vi "IMAQdx_grab_att - Kopie.vi"() -> ()   [LabVIEW 2015]
doc: "The Grab VI acquires images continuously and displays the images in an image control using low-level acquisition VIs. A grab is appropriate for high-speed applications in which you need to process only one image at a time."
uses:
  <vilib>/userdefined/High Color/IMAQdx.ctl
  <vilib>/vision/driver/IMAQdx.llb/IMAQdx Attribute Type.ctl
  <vilib>/vision/driver/IMAQdx.llb/IMAQdx Acquisition Mode.ctl
  <vilib>/vision/driver/IMAQdx.llb/IMAQdx Buffer Number Mode.ctl
  <vilib>/vision/driver/NI_Vision_Acquisition_Software.lvlib
  <resource>/objmgr/imaqdx.rc
  <vilib>/vision/NI_Vision_Development_Module.lvlib
panel:
  out "Exposure::Mode 2":u32(ring)=2 caption="Exposure::Mode" items=["Auto"=1, "Manual"=2]
  in  "String":string="um"
  out "output cluster":cluster{sgl, sgl}
  out "Last Mouse Position:All Elements":cluster{"X":i32, "Y":i32}
  in  "Gain::Value":i64 min=0 max=1728 step=1
  in  "Gain::Mode":u32(ring)=2 items=["Auto"=1, "Manual"=2]
  in  "Exposure::Value":dbl=0.0625 min=0.0 max=0.125
  in  "Exposure::Mode":u32(ring)=2 items=["Auto"=1, "Manual"=2]
  in  "Pixel Distances":T1={"X Step"=5.2, "Y Step"=5.2, "Unit"=enum."Micrometer"} {"Y Step" format="%.2f"; "X Step" format="%.2f"}
  out "Image Pixels (U8)":u8[][](array[numeric])
  out "error out":errorcluster
  out "Luminance Plane":T3(plugin-control)
  out "MinDBL":dbl
  out "MaxDBL":dbl
  out "Units":string
  in  "SetExpMode":enum16{"Dont use this!", "Auto", "Manual"}(ring)=enum."Auto"
  out "GetExpVal":dbl
  out "Attribute Information Array":T5(array[cluster])
  in  "InitExpVal":dbl
  out "IMAQdx Session":T6
  in  "Camera Name":refnum<k21>="cam0" caption="IMAQdx Session"
  out "Buffer Number":u32
  out "Image":T3(plugin-control)
  out "Frame Rate":dbl(knob) scale=0.0..20.0
  in  "Stop":bool
  # "Overview: Demonstrates how to acquire continuous images from a camera using low level acquisition functions.\nRequirements: Vision Acquisition Software\nInstructions:\n1. Select the Camera Name\n2. Run the VI"
  # "x /µm"
  # "y /µm"
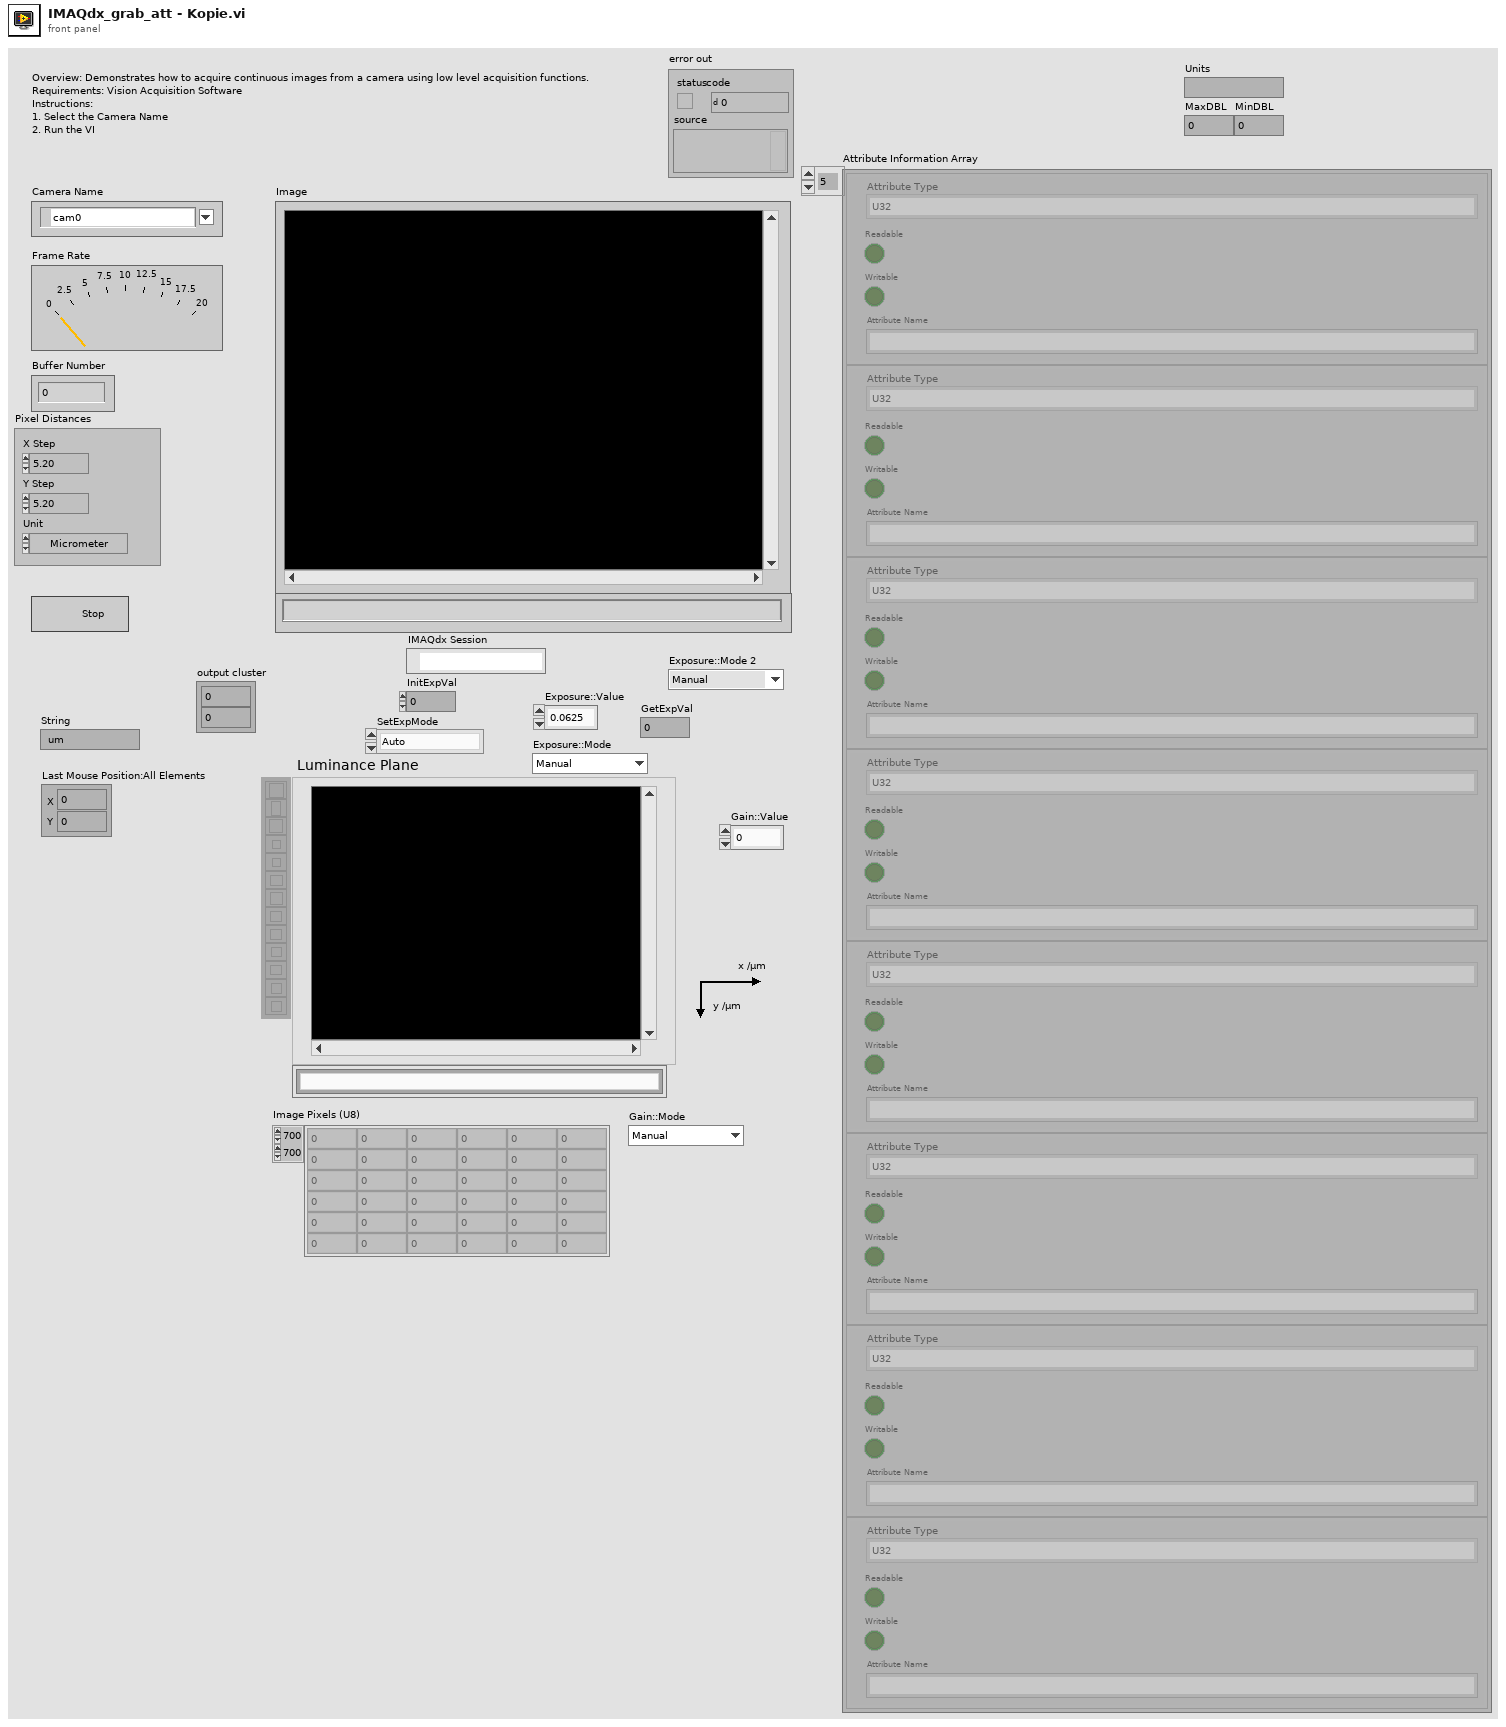
[diagram p1: front panel]
types:
  T1 = typedef "Simple Grid Descriptor" = cluster{"X Step":sgl, "Y Step":sgl, "Unit":T2}
  T2 = typedef "Image Unit" = enum32{"Undefined", "Angström", "Micrometer", "Millimeter", "Centimeter", "Meter", "Kilometer", "Microinch", "Inch", "Feet", "Nautical miles", "Standard miles", "Steps"}
  T3 = typedef "IMAQ Image.ctl" = refnum<image>
  T4 = typedef "NI_Vision_Acquisition_Software.lvlib/IMAQdx Attribute Type.ctl" = enum32{"U32", "I64", "DBL", "String", "Enum", "Bool", "Command"}
  T5 = cluster{"Attribute Type":T4, "Readable":bool, "Writable":bool, "Attribute Name":string}[]
  T6 = typedef "IMAQdx.ctl" = refnum<k21>
  T7 = typedef "Image Type" = u32
  T8 = typedef "NI_Vision_Acquisition_Software.lvlib/IMAQdx Acquisition Mode.ctl" = enum32{"One Shot", "Continuous"}
  T9 = typedef "NI_Vision_Acquisition_Software.lvlib/IMAQdx Buffer Number Mode.ctl" = enum32{"Next", "Last", "Buffer Number", "Every", "Last New"}
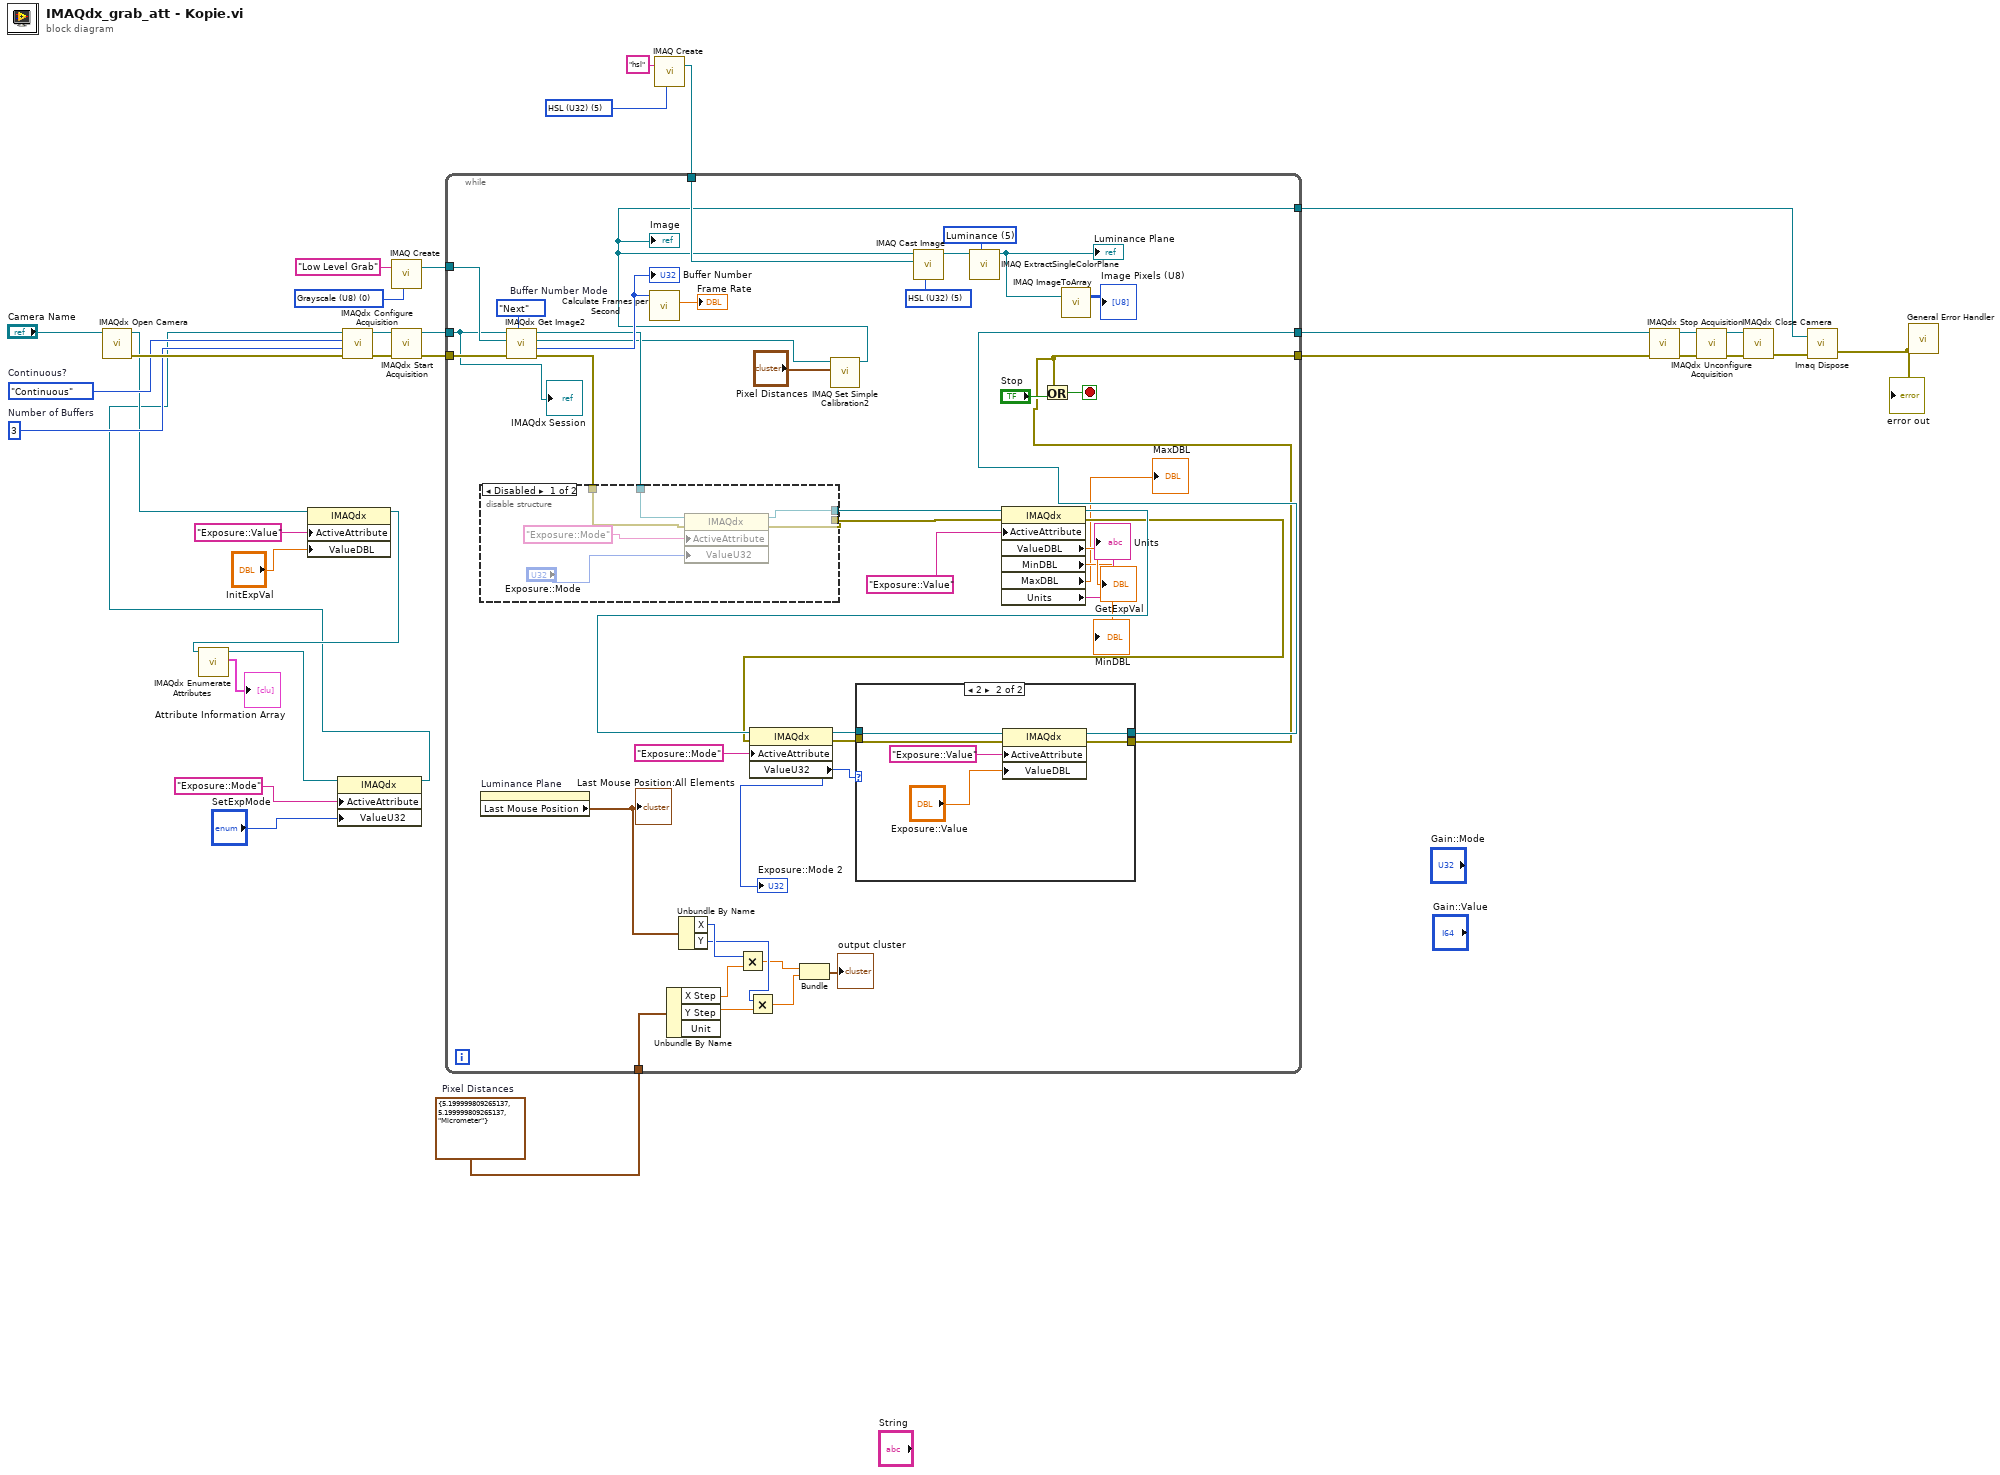
[diagram p0: block diagram]
diagram:
  w1 = T1 {"X Step"=5.2, "Y Step"=5.2, "Unit"=enum."Micrometer"}  # Pixel Distances
  w8 = T7 5 items=["Grayscale (U8)", "Grayscale (I16)", "Grayscale (SGL)", "Complex (CSG)", "RGB (U32)", "HSL (U32)", "RGB (U64)"] ("Image Type")
  w10 = T7 0 items=["Grayscale (U8)", "Grayscale (I16)", "Grayscale (SGL)", "Complex (CSG)", "RGB (U32)", "HSL (U32)", "RGB (U64)", "Grayscale (U16)"] ("Image Type")
  w26 = u32 3  # Number of Buffers
  w27 = IMAQdx_Acquisition_Mode."Continuous"  # Continuous?
  n1 = call <vilib>:"IMAQdx Open Camera.vi"("Session In"="Camera Name") -> ("error out"=w30:errorcluster, "Session Out"=w15:T6)  [unwired: 2 in, 7 out]
  n2 = property class="IMAQdx"(reference=w15, "ActiveAttribute"="Exposure::Value", "ValueDBL"="InitExpVal") -> (reference out=w12:T6)  [unwired: 1 in, 1 out]
  n3 = call <vilib>:"IMAQdx Enumerate Attributes.vi"("Session In"=w12) -> ("Attribute Information Array"=→"Attribute Information Array":T5, "Session Out"=w5:T6)  [unwired: 8 in, 1 out]
  n4 = property class="IMAQdx"(reference=w5, "ActiveAttribute"="Exposure::Mode", "ValueU32"="SetExpMode") -> (reference out=w4:T6)  [unwired: 1 in, 1 out]
  n5 = call <vilib>:"IMAQdx Configure Acquisition.vi"("error in"=w30, "Number of Buffers"=w26, "Continuous?"=w27, "Session In"=w4) -> ("error out"=w29:errorcluster, "Session Out"=w31:T6)  [unwired: 6 out]
  n6 = call "IMAQ Create"("Image Name"="Low Level Grab", "Image Type"=w10) -> ("New Image"=w33:T3)  [unwired: 2 in, 2 out]
  n7 = call <vilib>:"IMAQdx Start Acquisition.vi"("error in"=w29, "Session In"=w31) -> ("error out"=w28:errorcluster, "Session Out"=w2:T6)  [unwired: 8 out]
  n8 = call "IMAQ Create"("Image Name"="hsl", "Image Type"=w8) -> ("New Image"=w7:T3)  [unwired: 3 in, 1 out]
  n9 = while {
    tunnel: [w63] -> w24
    tunnel: w28 -> [w75]
    tunnel: w2 -> [w69]
    tunnel: [w62] -> w25
    tunnel: w33 -> [w74]
    tunnel: [w47] -> w16
    tunnel: w7 -> [w50]
    tunnel: w1 -> [w44]
    stop <- w76 stop-if-true
    w52 = 5 items=["Red", "Green", "Blue", "Hue", "Saturation", "Luminance", "Value", "Intensity"] ("Color Plane")
    w53 = T7 5 items=["Grayscale (U8)", "Grayscale (I16)", "Grayscale (SGL)", "Complex (CSG)", "RGB (U32)", "HSL (U32)", "RGB (U64)"] ("Image Type")
    w72 = IMAQdx_Buffer_Number_Mode."Next"  # Buffer Number Mode
    n10 = property on="Luminance Plane" class="ImageControl"() -> ("Last Mouse Position"=w43:cluster{"X":i32, "Y":i32})  [unwired: 2 in, 2 out]
    "Last Mouse Position:All Elements" <- w43
    n11 = call <vilib>:"IMAQdx Get Image2.vi"("Buffer Number Mode (Next)"=w72, "error in"=w75, "Image In"=w74, "Session In"=w69) -> ("error out"=w65:errorcluster, "Buffer Number Out"=w71:u32, "Image Out"=w46:T3, "Session Out"=w64:T6)  [unwired: 4 in]
    "Buffer Number" <- w71
    n12 = disable-structure shown="Disabled" {
      disable-tunnel: [w81 w84] -> w67
      disable-tunnel: [w80 w83] -> w66
      disable-tunnel: w65 -> [w79 w83]
      disable-tunnel: w64 -> [w78 w84]
      frame Disabled {
        n13 = property class="IMAQdx"(reference=w78, error in=w79, "ActiveAttribute"="Exposure::Mode", "ValueU32"="Exposure::Mode") -> (reference out=w81:T6, error out=w80:errorcluster)
      }
      frame Enabled {
      }
    }
    n14 = call <vilib>:"Calculate Frames per Second.vi"("Buffer Number"=w71) -> ("Processed Frames/s"=→"Frame Rate":dbl)  [unwired: 8 in, 2 out]
    n15 = Unbundle By Name(w44) -> ("X Step"=w41:sgl, "Y Step"=w39:sgl)  [unwired: 1 out]
    n16 = Unbundle By Name(w43) -> ("X"=w42:i32, "Y"=w40:i32)
    n17 = Multiply(x=w42, y=w41) -> (x*y=w37:sgl)
    n18 = Multiply(x=w40, y=w39) -> (x*y=w38:sgl)
    n19 = Bundle(w37, w38) -> (→"output cluster":cluster{sgl, sgl})  [unwired: 1 in]
    n20 = call "IMAQ Set Simple Calibration2"("Pixel Distances"="Pixel Distances", "Image"=w46) -> ("Calibration Template Image"=w47:T3)  [unwired: 8 in, 1 out]
    "Image" <- w47
    n21 = call "IMAQ Cast Image"("Image Type"=w53, "Image Dst"=w50, "Image Src"=w47) -> ("Image Dst Out"=w51:T3)  [unwired: 7 in, 1 out]
    n22 = call "IMAQ ExtractSingleColorPlane"("Color Plane"=w52, "Image Src"=w51) -> ("Image Dst Out"=w45:T3)  [unwired: 8 in, 1 out]
    "Luminance Plane" <- w45
    n23 = property class="IMAQdx"(reference=w67, error in=w66, "ActiveAttribute"="Exposure::Value") -> (reference out=w59:T6, error out=w58:errorcluster, "ValueDBL"=→"GetExpVal":dbl, "MinDBL"=→"MinDBL":dbl, "MaxDBL"=→"MaxDBL":dbl, "Units"=→"Units":string)
    n24 = property class="IMAQdx"(reference=w59, error in=w58, "ActiveAttribute"="Exposure::Mode") -> (reference out=w57:T6, error out=w56:errorcluster, "ValueU32"=w34:u32)
    "Exposure::Mode 2" <- w34
    n25 = case shown="2" w34 {
      tunnel: w57 -> [w86 w91]
      tunnel: w56 -> [w85 w90]
      tunnel: [w86 w89] -> w63
      tunnel: [w85 w88] -> w62
      frame 1, Default {
      }
      frame 2 {
        n26 = property class="IMAQdx"(reference=w91, error in=w90, "ActiveAttribute"="Exposure::Value", "ValueDBL"="Exposure::Value") -> (reference out=w89:T6, error out=w88:errorcluster)
      }
    }
    n27 = Or(x=w62, y="Stop") -> (x .or. y?=w76:bool)
    n28 = call "IMAQ ImageToArray"("Image"=w45) -> ("Image Pixels (U8)"=→"Image Pixels (U8)":u8[][])  [unwired: 3 in, 4 out]
    "IMAQdx Session" <- w69
  }
  n29 = call <vilib>:"IMAQdx Stop Acquisition.vi"("error in"=w25, "Session In"=w24) -> ("error out"=w20:errorcluster, "Session Out"=w21:T6)  [unwired: 8 out]
  n30 = call <vilib>:"IMAQdx Unconfigure Acquisition.vi"("error in"=w20, "Session In"=w21) -> ("error out"=w23:errorcluster, "Session Out"=w22:T6)  [unwired: 8 out]
  n31 = call <vilib>:"IMAQdx Close Camera.vi"("error in"=w23, "Session In"=w22) -> ("error out"=w19:errorcluster)  [unwired: 9 out]
  n32 = call "Imaq Dispose"("Image"=w16, "error in (no error)"=w19) -> ("error out"=w18:errorcluster)  [unwired: 4 in]
  "error out" <- w18
  n33 = call <vilib>:"General Error Handler.vi"("error in (no error)"=w18) -> ()  [unwired: 2 in, 13 out]
